vi "Read in XML.vi"(8 "error in":errorcluster, 11 "Path to XML":path=path "D:/Software/Optical-Prime") -> (0 "error out":errorcluster, 3 "OpticalPrime Ctrls For Saving":T1={"Time Stamp"={"date string"="", "time string"=""}, "Exp Params"={"Experiment Type"="Time Series", "Experiment Name"="Experiment_1", "ExpPath"=path "D:/Data", "Save As"="TIFF", "TSFrames"=1000, "TSfps"=1.0, "Streaming"=TRUE, "tdms ref"=refnum, "frame #"=0, "Full Path"=path "", "PeakOnQueue"=FALSE}, "Ventus Controls"={"Ventus Power"=0.0, "Open Serial"=FALSE, "VISA Refnum"=""}, "Camera Controls"={"Exposure Time (ms)"=27, "cam0 Session"="", "Camera ROI"={"Width"=0, "Height"=0, "Offset X"=0, "Offset Y"=0}, "Command"=""}, "Spot Params"=[], "SLM Parameters"={"Width"=0.0, "Height"=0.0, "Board ID"=0, "Centre Y"=0.0, "Centre X"=0.0}} {"Spot Params"."Z" format="%_4g"; "Spot Params"."Y" format="%_4g"; "Spot Params"."X" format="%_4g"; "Spot Params"."Phase" format="%_4g"; "Spot Params"."Intensity" format="%_4g"; "Camera Controls"."Camera ROI"."Offset Y" max=2046 step=2; "Camera Controls"."Camera ROI"."Offset X" max=2044 step=4; "Camera Controls"."Camera ROI"."Height" min=2 max=2048 step=2; "Camera Controls"."Camera ROI"."Width" min=4 max=2048 step=4; "Camera Controls"."Exposure Time (ms)" min=27 max=500 step=1 scale=27.0..500.0; "SLM Parameters"."Centre X" format="%.3g"; "SLM Parameters"."Centre Y" format="%.3g"; "Ventus Controls"."Ventus Power" min=0.0 max=100.0 step=0.1 scale=0.0..100.0; "Exp Params"."TSFrames" min=1 step=1; "Exp Params"."TSfps" min=0.001 max=90.0 step=0.001 format="%_4g"})   [LabVIEW 2020]
uses:
  _controls/OpticalPrime Ctrls For Saving.ctl
  _controls/Exp Params.ctl
  _controls/Ventus Control.ctl
  _controls/xiCam.ctl
  <vilib>/userDefined/High Color/IMAQdx.ctl
  _controls/Spot Params.ctl
  _controls/PCIe SLM params.ctl
  <vilib>/Utility/xml.llb/Read From XML File(string).vi
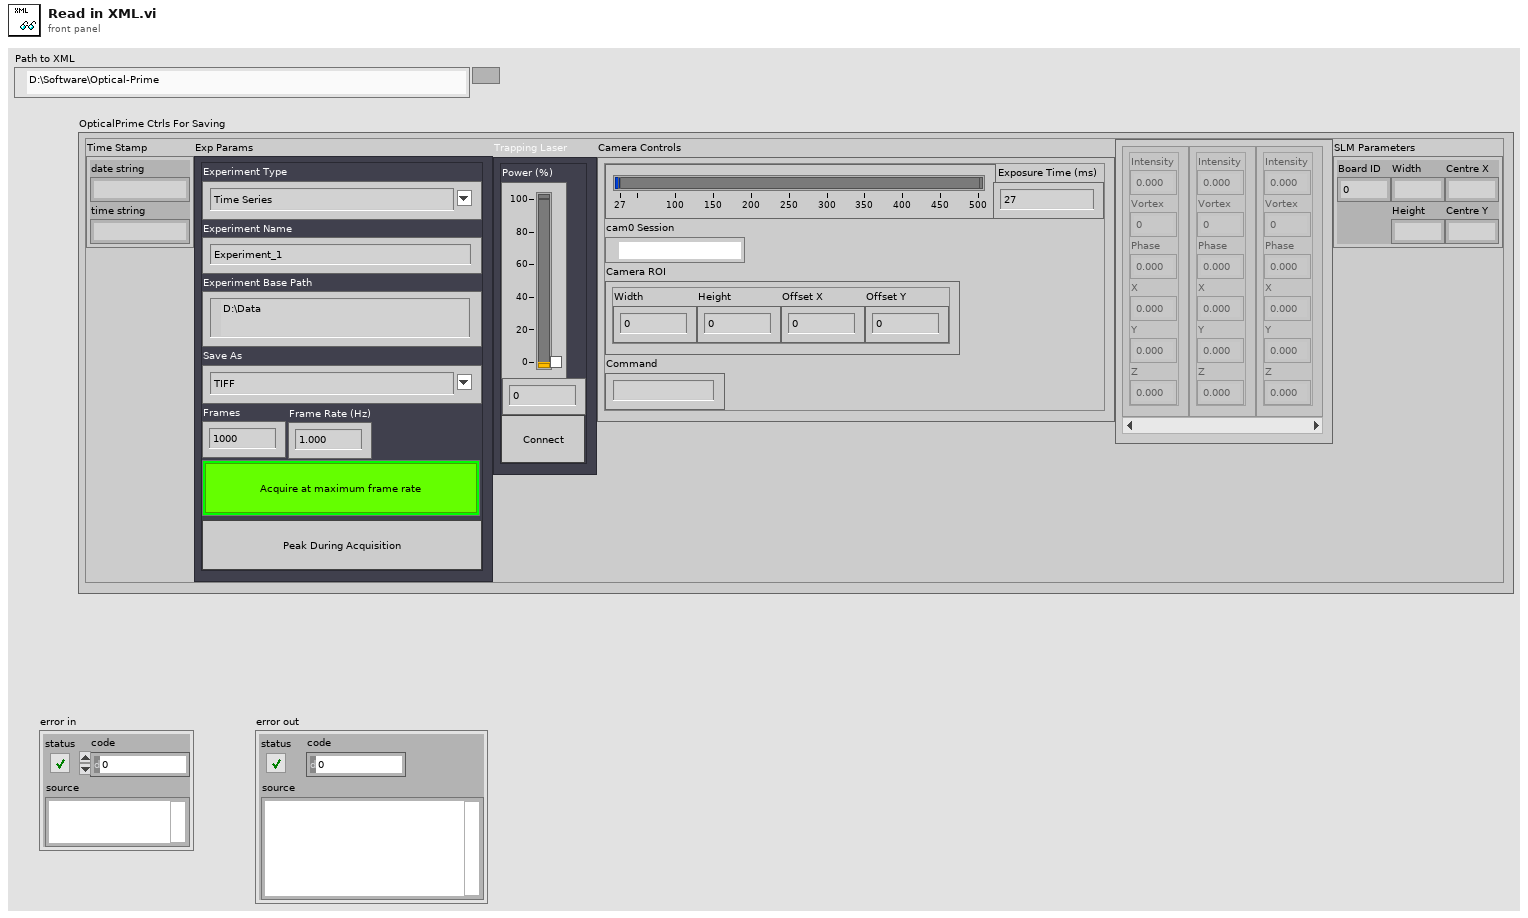
[diagram p1: front panel]
types:
  T1 = typedef "OpticalPrime Ctrls For Saving.ctl" = cluster{"Time Stamp":cluster{"date string":string, "time string":string}, "Exp Params":T2, "Ventus Controls":T3, "Camera Controls":T4, "Spot Params":T6, "SLM Parameters":T7}
  T2 = typedef "Exp Params.ctl" = cluster{"Experiment Type":string, "Experiment Name":string, "ExpPath":path, "Save As":string, "TSFrames":i32, "TSfps":dbl, "Streaming":bool, "tdms ref":refnum<k34>, "frame #":i64, "Full Path":path, "PeakOnQueue":bool}
  T3 = typedef "Ventus Control.ctl" = cluster{"Ventus Power":dbl, "Open Serial":bool, "VISA Refnum":refnum<visa-resource-name>}
  T4 = typedef "xiCam.ctl" = cluster{"Exposure Time (ms)":u32, "cam0 Session":T5, "Camera ROI":cluster{"Width":u32, "Height":u32, "Offset X":u32, "Offset Y":u32}, "Command":string}
  T5 = typedef "IMAQdx.ctl" = refnum<k21>
  T6 = typedef "Spot Params.ctl" = cluster{"Intensity":dbl, "Vortex":dbl, "Phase":dbl, "X":dbl, "Y":dbl, "Z":dbl}[]
  T7 = typedef "PCIe SLM params.ctl" = cluster{"Width":dbl, "Height":dbl, "Board ID":i32, "Centre Y":dbl, "Centre X":dbl}
  T8 = cluster{"Time Stamp":cluster{"date string":string, "time string":string}, "Exp Params":T2, "Ventus Controls":T3, "Camera Controls":T4, "Spot Params":T6, "SLM Parameters":T7}
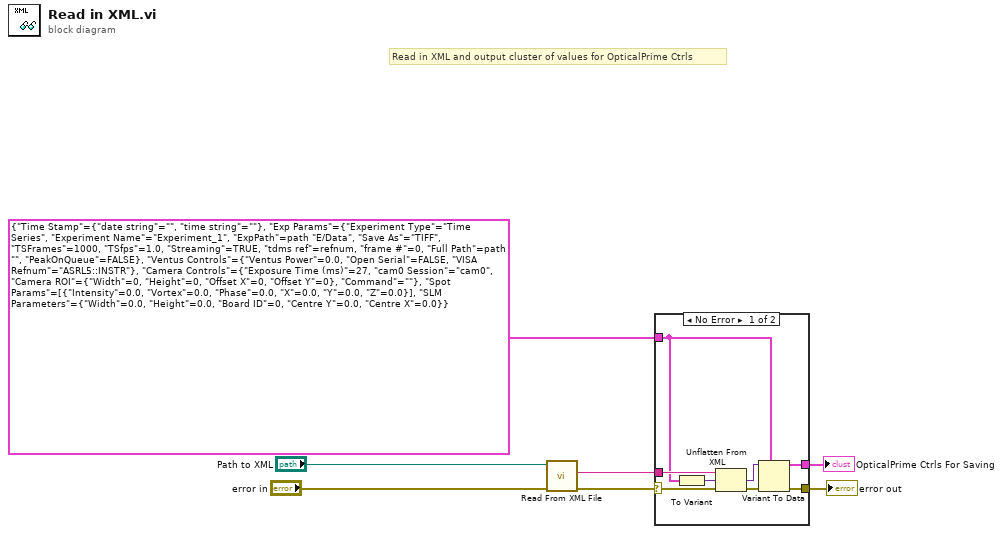
[diagram p0: block diagram]
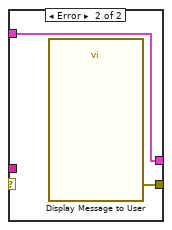
[diagram p2: hidden frame]
diagram:
  # "Read in XML and output cluster of values for OpticalPrime Ctrls"
  n1 = call-poly <vilib>:"Read From XML File.vi"("error in (no error)"="error in", "XML File Path"="Path to XML") -> ("error out"=w4:errorcluster, "XML Elements"=w5:string)  [unwired: 7 in, 1 out]
  n2 = case shown="No Error" w4 {
    selector: w4 -> [w11 _]
    tunnel: [w15 w17] -> w6
    tunnel: [w8 w16] -> w2
    tunnel: w5 -> [w13 _]
    tunnel: T8 {"Time Stamp"={"date string"="", "time string"=""}, "Exp Params"={"Experiment Type"="Time Series", "Experiment Name"="Experiment_1", "ExpPath"=path "E:/Data", "Save As"="TIFF", "TSFrames"=1000, "TSfps"=1.0, "Streaming"=TRUE, "tdms ref"=refnum, "frame #"=0, "Full Path"=path "", "PeakOnQueue"=FALSE}, "Ventus Controls"={"Ventus Power"=0.0, "Open Serial"=FALSE, "VISA Refnum"="ASRL5::INSTR"}, "Camera Controls"={"Exposure Time (ms)"=27, "cam0 Session"="cam0", "Camera ROI"={"Width"=0, "Height"=0, "Offset X"=0, "Offset Y"=0}, "Command"=""}, "Spot Params"=[{"Intensity"=0.0, "Vortex"=0.0, "Phase"=0.0, "X"=0.0, "Y"=0.0, "Z"=0.0}], "SLM Parameters"={"Width"=0.0, "Height"=0.0, "Board ID"=0, "Centre Y"=0.0, "Centre X"=0.0}} ("OpticalPrime Ctrls For Saving") -> [w9 w16]
    frame No Error {
      n3 = To Variant(anything=w9) -> (Variant=w14:variant)
      n4 = Unflatten From XML(xml string=w13, type=w14, error in (no error)=w11) -> (value=w12:variant, error out=w10:errorcluster)
      n5 = Variant To Data(error in=w10, type=w9, Variant=w12) -> (data=w8:T8, error out=w15:errorcluster)
    }
    frame Error {
      n6 = call "Display Message to User"() -> ("error out"=w17:errorcluster)  [unwired: 10 in, 1 out]
    }
  }
  "error out" <- w6
  "OpticalPrime Ctrls For Saving" <- w2
